vi "process_shutter.vi"(6 "error in (no error)":errorcluster) -> (0 "error out":errorcluster)   [LabVIEW 2010]
uses:
  typedefs/control_shutter_enum.ctl
  <vilib>/DAQmx/write.llb/DAQmx Write (Digital Bool 1Line 1Point).vi
  <vilib>/DAQmx/create/channels.llb/DAQmx Create Channel (DO-Digital Output).vi
  <vilib>/daqmx/miscellaneous.llb/DAQmx Fill In Error Info.vi
panel:
  out "Shutter":bool
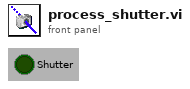
[diagram p1: front panel]
types:
  T1 = typedef "control_shutter_enum.ctl" = enum16{"Init", "Open", "Close", "Quit"}
  T2 = cluster{"Control shutter enum":T1, "variant":variant}
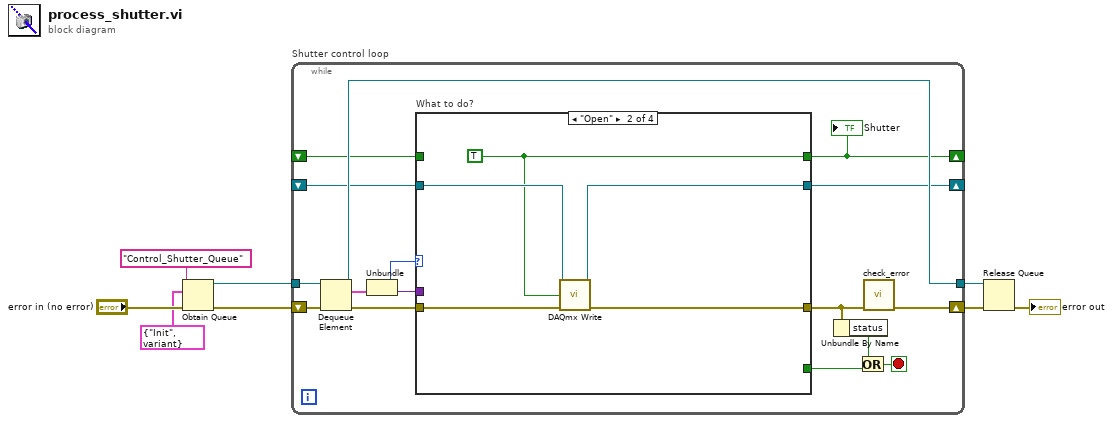
[diagram p0: block diagram]
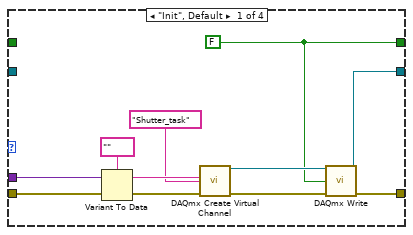
[diagram p2: hidden frame]
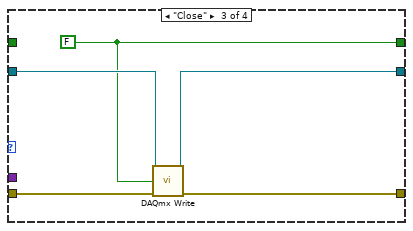
[diagram p3: hidden frame]
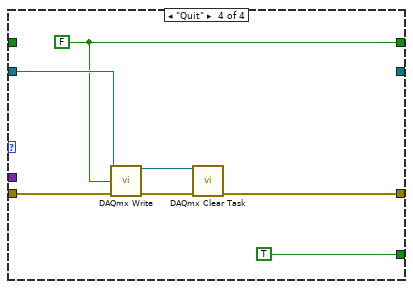
[diagram p4: hidden frame]
diagram:
  n1 = Obtain Queue(name (unnamed)="Control_Shutter_Queue", element data type=T2 {"Control shutter enum"=enum."Init", "variant"=variant}, error in (no error)="error in (no error)") -> (queue out=w2:refnum<queue>, error out=w1:errorcluster)  [unwired: 2 in, 1 out]
  n2 = while "Shutter control loop" {
    shift-right: [w9] -> w3
    shift-left: w1 -> [w23]
    tunnel: w2 -> [w24]
    tunnel: [w15] -> w5
    shift-right: [w14] -> _
    shift-left: _ -> [w13]
    shift-right: [w12] -> _
    shift-left: _ -> [w11]
    stop <- w17 stop-if-true
    n3 = Dequeue Element(queue=w24, error in (no error)=w23) -> (queue out=w15:refnum<queue>, element=w22:T2, error out=w19:errorcluster)  [unwired: 1 in, 1 out]
    n4 = Unbundle(w22) -> ("Control shutter enum"=w21:T1, "variant"=w20:variant)
    n5 = case "What to do?" shown="\"Open\"" w21 {
      tunnel: w20 -> [w35 _ _ _]
      tunnel: w19 -> [w25 w37 w42 w50]
      tunnel: [w30 w40 w45 w51] -> w10
      tunnel: [_ _ _ TRUE] -> w16
      tunnel: [w28 w36 w41 _] -> w14
      tunnel: w13 -> [_ w39 w44 w48]
      tunnel: [w27 w38 w43 w46] -> w12
      tunnel: w11 -> [_ _ _ _]
      frame "Init", Default {
        w27 = FALSE ("data")
        n6 = Variant To Data(error in=w25, Variant=w35, type=tag "" ("Shutter channel")) -> (error out=w34:errorcluster, data=w33:tag)
        n7 = call-poly <vilib>:"DAQmx Create Virtual Channel.vi"("lines"=w33, "name to assign"="Shutter_task", "error in"=w34) -> ("task out"=w29:refnum<k21>, "error out"=w31:errorcluster)  [unwired: 11 in]
        n8 = call-poly <vilib>:"DAQmx Write.vi"("task/channels in"=w29, "data"=w27, "error in"=w31) -> ("task out"=w28:refnum<k21>, "error out"=w30:errorcluster)  [unwired: 10 in, 1 out]
      }
      frame "Open" {
        w38 = TRUE
        n9 = call-poly <vilib>:"DAQmx Write.vi"("task/channels in"=w39, "data"=w38, "error in"=w37) -> ("task out"=w36:refnum<k21>, "error out"=w40:errorcluster)  [unwired: 10 in, 1 out]
      }
      frame "Close" {
        w43 = FALSE
        n10 = call-poly <vilib>:"DAQmx Write.vi"("task/channels in"=w44, "data"=w43, "error in"=w42) -> ("task out"=w41:refnum<k21>, "error out"=w45:errorcluster)  [unwired: 10 in, 1 out]
      }
      frame "Quit" {
        w46 = FALSE ("data")
        n11 = call-poly <vilib>:"DAQmx Write.vi"("task/channels in"=w48, "data"=w46, "error in"=w50) -> ("task out"=w47:refnum<k21>, "error out"=w49:errorcluster)  [unwired: 10 in, 1 out]
        n12 = call <vilib>:"DAQmx Clear Task.vi"("task in"=w47, "error in"=w49) -> ("error out"=w51:errorcluster)  [unwired: 13 in]
      }
    }
    "Shutter" <- w12
    n13 = Unbundle By Name(w10) -> ("status"=w18:bool)
    n14 = Or(x=w18, y=w16) -> (x .or. y?=w17:bool)
    n15 = call "check_error.vi"("error in"=w10) -> ("error out"=w9:errorcluster)  [unwired: 10 in]
  }
  n16 = Release Queue(queue=w5, error in (no error)=w3) -> (error out=→"error out":errorcluster)  [unwired: 1 in, 2 out]
